vi "HEX to ASCII.vi"(1 "String in HEX":string) -> (0 "String in ASCII":string)   [LabVIEW 2015]
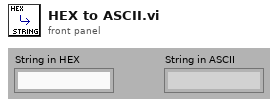
[diagram p1: front panel]
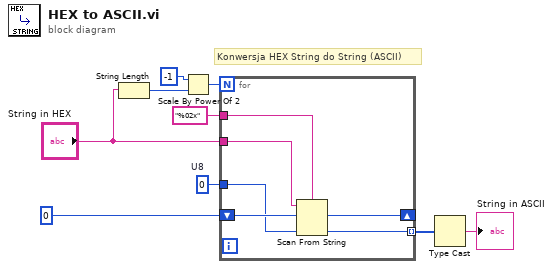
[diagram p0: block diagram]
diagram:
  w3 = u8 0  # U8
  # "Konwersja HEX String do String (ASCII)"
  n1 = String Length(string="String in HEX") -> (length=w6:i32)
  n2 = Scale By Power Of 2(n=-1, x=w6) -> (x*2^n=w8:i32)
  n3 = for {
    N: w8 -> [_]
    shift-right: [w14] -> _
    shift-left: u32 0 -> [w15]
    tunnel: "String in HEX" -> [w13]
    tunnel: w3 -> [w12]
    tunnel: [w11] -> w4 mode=indexing
    tunnel: "%02x" ("format string") -> [w10]
    n4 = Scan From String(format string=w10, input string=w13, initial scan location=w15, default 1=w12) -> (offset past scan=w14:u32, output 1=w11:u8)  [unwired: 1 in, 2 out]
  }
  n5 = Type Cast(x=w4) -> (*(type *) &x=→"String in ASCII":string)  [unwired: 1 in]
